vi "Pulse Attribute, Record Results.vi"(7 "step name":string="Pulse Attribute Results", 8 "error in":errorcluster, 9 "test case":T2, 10 "results":T1[](array[typedef])=[{"Label"="Stim Amp (mA)", "Value"=nan}, {"Label"="Stim Pulse Width (us)", "Value"=nan}, {"Label"="Interphase Delay (us)", "Value"=nan}, {"Label"="Recvy Amp (mA)", "Value"=nan}, {"Label"="Recvy Pulse Width (us)", "Value"=nan}, {"Label"="Frequency (Hz)", "Value"=nan}, {"Label"="Period Jitter (us rms)", "Value"=nan}] {"Value" format="%#.3f"}, 11 "Sequence Context":refnum<k7>) -> (0 "error out":errorcluster, 3 "Sequence Context dup":refnum<k7>)   [LabVIEW 2010]
doc: "This function transfers a single Compare Data Test (CDT) record to the current TestStand sequence step."
uses:
  Active Output Test Cases.ctl
  Generic/Waveform Attribute/Waveform Attribute Cluster.ctl
panel:
  in  "Acceptance Criteria":string[][](table) caption="Table 1"
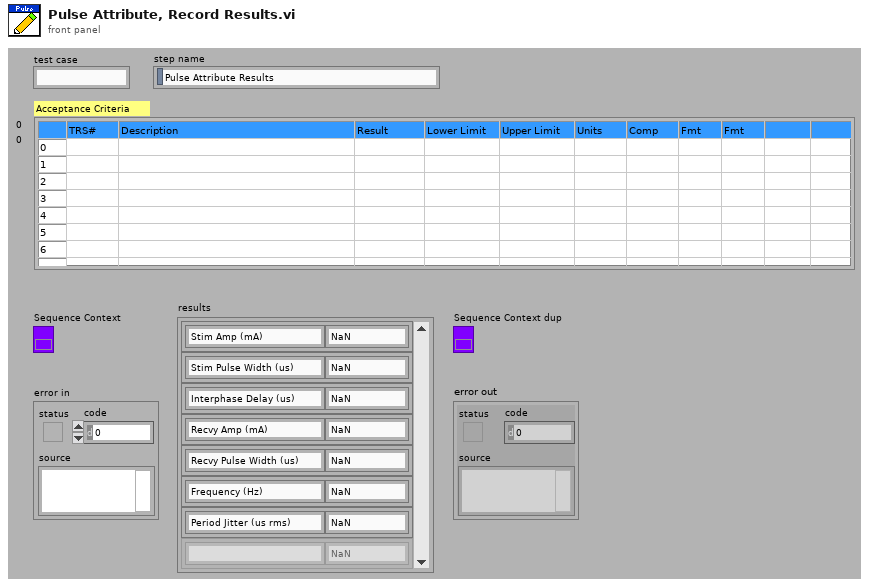
[diagram p1: front panel]
types:
  T1 = typedef "Waveform Attribute Cluster.ctl" = cluster{"Label":string, "Value":dbl}
  T2 = typedef "Active Output Test Cases.ctl" = string
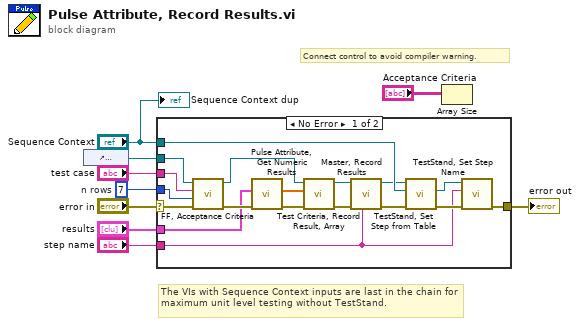
[diagram p0: block diagram]
diagram:
  w1 = 7  # n rows
  # "The VIs with Sequence Context inputs are last in the chain for maximum unit level testing without TestStand."
  # "Connect control to avoid compiler warning."
  n1 = control-ref of="Acceptance Criteria"() -> (w4:refnum<vi>)
  n2 = case shown="No Error" "error in" {
    selector: "error in" -> [w21 w28]
    tunnel: [w19 w28] -> w9
    tunnel: "Sequence Context" -> [w18 _]
    tunnel: "test case" -> [w16 _]
    tunnel: w4 -> [w22 _]
    tunnel: "results" -> [w24 _]
    tunnel: "step name" -> [w10 _]
    tunnel: w1 -> [w15 _]
    frame No Error {
      n3 = call "FF, Acceptance Criteria.vi"("error in"=w21, "n rows"=w15, "test case"=w16, "Tbl Refnum"=w22) -> ("error out"=w26:errorcluster, "Tbl Refnum out"=w27:refnum<vi>)  [unwired: 6 in]
      n4 = call "Pulse Attribute, Get Numeric Results.vi"("error in"=w26, "results"=w24) -> ("error out"=w25:errorcluster, "numeric values"=w23:dbl[])  [unwired: 4 in]
      n5 = call "Test Criteria, Record Result, Array.vi"("error in"=w25, "Results"=w23, "Tbl Refnum"=w27) -> ("error out"=w14:errorcluster, "Tbl Refnum out"=w12:refnum<vi>)  [unwired: 6 in, 1 out]
      n6 = call "Master, Record Results.vi"("step name"=w10, "error in"=w14, "Tbl Refnum"=w12) -> ("error out"=w13:errorcluster, "Tbl Refnum dup"=w11:refnum<vi>)  [unwired: 7 in]
      n7 = call "TestStand, Set Step from Table.vi"("error in"=w13, "Sequence Context"=w18, "Tbl Refnum"=w11) -> ("error out"=w20:errorcluster, "Sequence Context Out"=w17:refnum<k7>)  [unwired: 6 in, 1 out]
      n8 = call "TestStand, Set Step Name.vi"("error in"=w20, "Step Name"=w10, "Sequence Context"=w17) -> ("error out"=w19:errorcluster)  [unwired: 7 in, 1 out]
    }
    frame Error {
    }
  }
  "error out" <- w9
  n9 = Array Size(array="Acceptance Criteria") -> ()  [unwired: 1 out]
  "Sequence Context dup" <- "Sequence Context"
